vi "解析对应路径的PID.vi"(8 "error in (no error)":errorcluster caption="错误输入（无错误）", 9 "appname":string="平台数据传输系统.exe", 10 "Path":string="C:\\LabVIEW Project\\builds\\NEW平台数据传输系统 - 副本\\平台数据传输系统.exe", 11 "输入":string) -> (0 "error out":errorcluster caption="错误输出", 2 "同名app个数":i32, 3 "PID":string)   [LabVIEW 2016, in "自动更新.lvlib"]
panel:
  out "已删除元素的数组子集":string[](array[string])
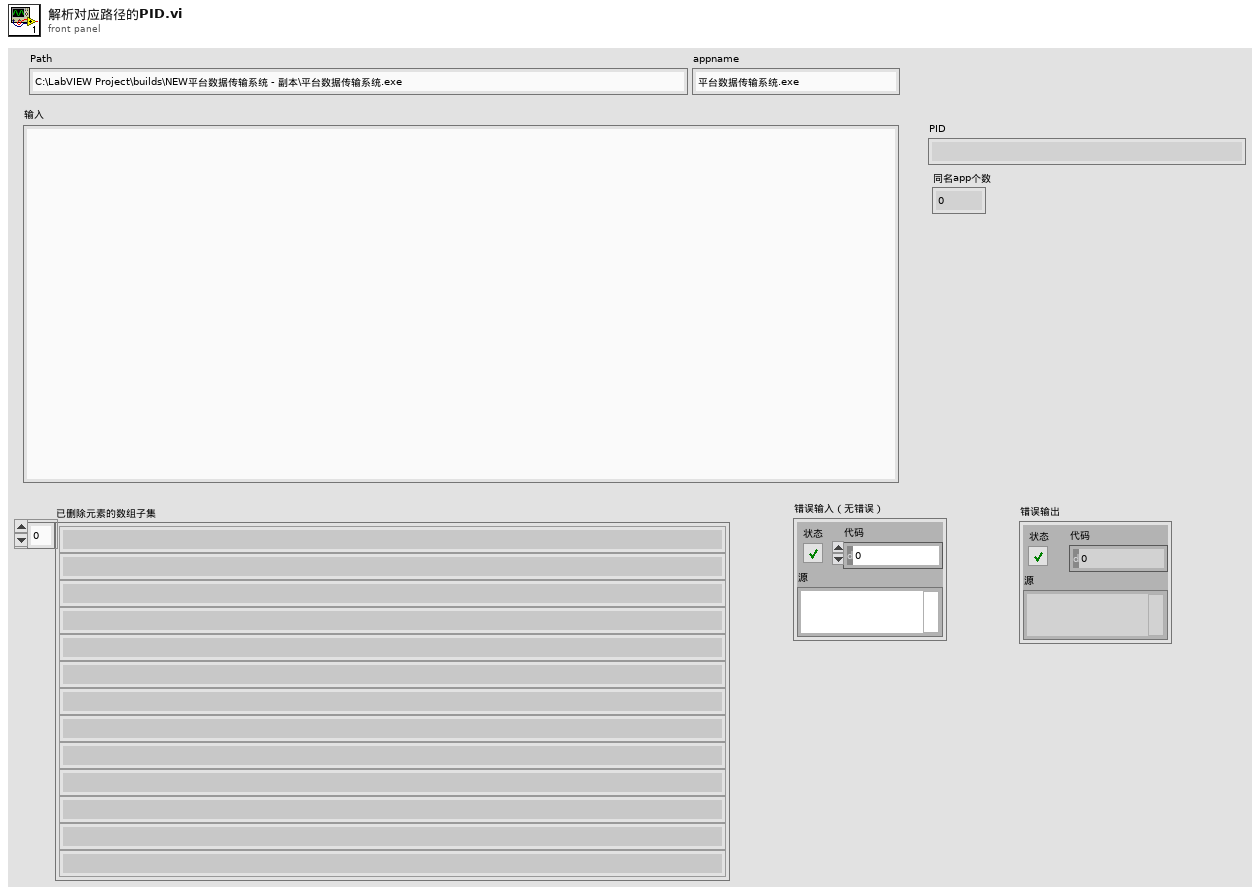
[diagram p1: front panel]
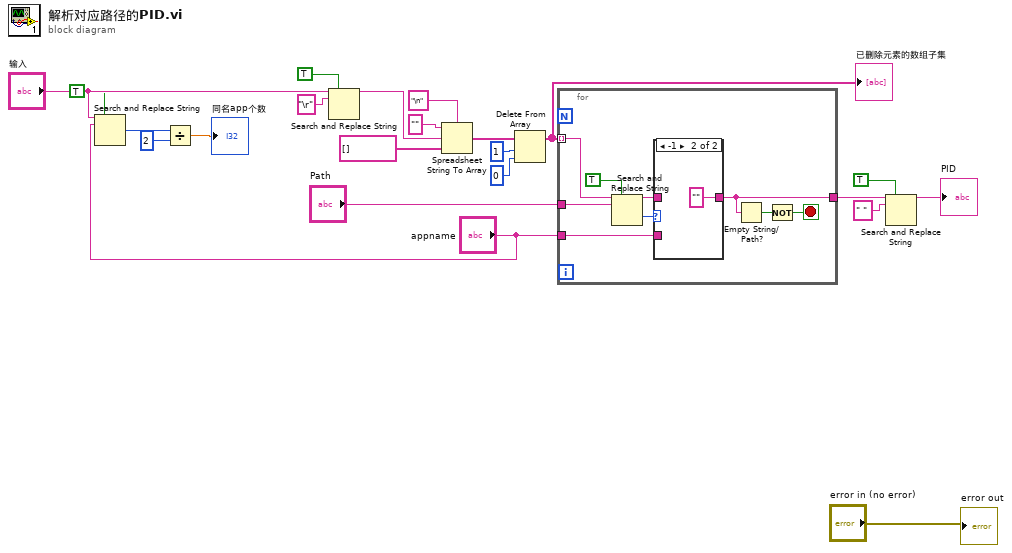
[diagram p0: block diagram]
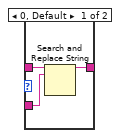
[diagram p2: hidden frame]
diagram:
  n1 = Search and Replace String(replace all?=TRUE ("替换全部？(F)"), input string="输入", search string="appname") -> (number of replacements=w3:i32)  [unwired: 5 in, 3 out]
  n2 = Divide(x=w3, y=2) -> (x/y=→"同名app个数":dbl)
  n3 = Search and Replace String(replace all?=TRUE ("替换全部？(F)"), input string="输入", search string="\r" ("搜索字符串")) -> (result string=w18:string)  [unwired: 5 in, 3 out]
  n4 = Spreadsheet String To Array(delimiter (Tab)="\n" ("分隔符(Tab)"), format string="" ("格式字符串"), spreadsheet string=w18, array type (2D Dbl)=string[] []) -> (array=w15:string[])
  n5 = Delete From Array(array=w15, length=1 ("长度"), index=0 ("索引")) -> (array with subset deleted=w12:string[])  [unwired: 1 out]
  "已删除元素的数组子集" <- w12
  n6 = for {
    tunnel: "appname" -> [w27]
    tunnel: "Path" -> [w31]
    tunnel: [w25] -> w9
    tunnel: w12 -> [w26] mode=indexing
    stop <- w23 stop-if-true
    n7 = Search and Replace String(replace all?=TRUE ("替换全部？(F)"), input string=w26, search string=w31) -> (result string=w28:string, offset past replacement=w29:i32)  [unwired: 5 in, 2 out]
    n8 = case shown="-1" w29 {
      tunnel: w28 -> [w34 _]
      tunnel: [w33 "" ("result string")] -> w25
      tunnel: w27 -> [w32 _]
      frame 0, Default {
        n9 = Search and Replace String(input string=w34, search string=w32) -> (result string=w33:string)  [unwired: 6 in, 3 out]
      }
      frame -1 {
      }
    }
    n10 = Empty String/Path?(string/path=w25) -> (empty?=w24:bool)
    n11 = Not(x=w24) -> (.not. x?=w23:bool)
  }
  n12 = Search and Replace String(replace all?=TRUE ("替换全部？(F)"), input string=w9, search string=" " ("搜索字符串")) -> (result string=→"PID":string)  [unwired: 5 in, 3 out]
  "error out" <- "error in (no error)"
